vi "IV analysis.vi"() -> ()   [LabVIEW 2020]
uses:
  <userlib>/Levylab/LV to ITX/Data/Typedefs/File Type--enum.ctl
  <userlib>/Levylab/XY Utilities/subVIs/Savitsky Golay Filter (single).vi
  <userlib>/Levylab/XY Utilities/subVIs/Difference Quotient (single).vi
  <userlib>/Levylab/XY Utilities/xy_utilities.lvlib
  data-analysis-megan/Retrieve and Visualize/Retrieve and Visualize.lvclass
  <userlib>/Levylab/LV to ITX/Data/Data.lvclass
panel:
  in  "start (length of curve)":i32
  in  "length of curve":i32
  in  "side points 2T":i32
  in  "side points 4T":i32
  in  "Interval Units":enum16{"Points", "Data"}(ring)
  in  "Window [h]":dbl=250.0 min=2.0
  in  "Tab Control":T1(tab)
  in  "index":T2
  in  "File or Folder Path":path=path "C:/Users/voodoo/Desktop/IV_separat_Vsgsweep_2fields_Vbg-2.8V"
  in  "decimate files":i32=1
  in  "offset":i32
  in  "length":i32=1
  in  "File Type":T3
  out "Comments":string="Device: \r  Device Name: SA40178.20210125\r  Computer: KHOLEK\r  User: Aditi\r  Instrument: MNK\r  Description: |\r        devices:\r        \r        1. 80x80um rectangle\r        2. hash: 200 horizontal and vertical lines 400nm apart\r        3. hash structures: 400, 200nm apart horizontal and vertical lines\r\rExperiment: \r  Time: 2021-02-01T16:02:55\r  Description: |\r     IV measurements at 0T\r     - Sweep priority 0: +x gate from -10V to 10V in steps of 1V (-x 10 to -10)\r     - priority 1:+y gate from -10V to 10V in steps of 1V (-y 10 to -10)\r    - 5s wait\r     - 1 IV curves at each Vsg\r     - KH channel 17,18,19,20: leads 3,8,15,27\r    Vbg = lead 26: 0V\r    T: 20mK\r    \r    \r    400nm periodicity mesh\r    \r    KH channel 2,1: leads 5,4 , current mode, 5k resistor, 1000x gain\r    lead 5: 10mV ac+ 0uV dc bias, 0.02 Hz\r    KH channel 3,4: V1+/-: 6,7 1000x gain\r    \r    rectangle\r    \r    KH channel 5,8: leads 9,13 , current mode, 5k resistor, 1000x gain\r     lead 9: 10mV ac+ 0uV dc bias, 0.02 Hz\r     KH channel 6,7: V1+/-: 11,12 1000x gain\r    \r    \r    200nm periodicity mesh\r    \r    KH channel 12,11: leads 21,20 , current mode, 5k resistor, 1000x gain\r    lead 21: 10mV ac+ 180uV dc bias, 0.02 Hz\r    KH channel 9,10: V1+/-: 16,17 1000x gain\r    \r    line filter on in lockin\r    decimating factor: 5\r\rSweep: \r- Loop1: [Lockin Bias, 10.000000]\r- Loop2: [Lockin Bias, 10.000000]\r- Loop3: [OFF, 0.000000]\r- Loop4: [OFF, 0.000000]\r\rWiring: \r- Electrode 4: Lockin 1, I2, KH1 Channel 1, Differential, 1000x, 5k Ohms\r- Electrode 5: Lockin 2, I2, KH1 Channel 2, Differential, 1000x, 5k Ohms\r- Electrode 6: Lockin 3, V2, KH1 Channel 3, SE+ (-gnd), 1000x, Open\r- Electrode 7: Lockin 4, V2, KH1 Channel 4, SE+ (-gnd), 1000x, Open\r- Electrode 9: Lockin 5, I2, KH1 Channel 5, Differential, 1000x, 5k Ohms\r- Electrode 11: Lockin 6, V2, KH1 Channel 6, SE+ (-gnd), 1000x, Open\r- Electrode 12: Lockin 7, V2, KH1 Channel 7, SE+ (-gnd), 1000x, Open\r- Electrode 13: Lockin 8, I2, KH1 Channel 8, Differential, 1000x, 5k Ohms\r- Electrode 16: Lockin 9, V1+, KH2 Channel 1, SE+ (-gnd), 1000x, Open\r- Electrode 17: Lockin 10, V1-, KH2 Channel 2, SE+ (-gnd), 1000x, Open\r- Electrode 20: Lockin 11, I-, KH2 Channel 3, Differential, 1000x, 5k Ohms\r- Electrode 21: Lockin 12, I+, KH2 Channel 4, Differential, 1000x, 5k Ohms\r- Electrode 1: Lockin 13, Vsg, KH2 Channel 5, Differential, 1000x, 50k Ohms\r\rLockin: \r  AO: \r  - AO 1: amp = 0.000 mV, DC = 0.000 mV, f = 0.02 Hz, phi = 0.00°, Triangle\r  - AO 2: amp = 10.000 mV, DC = 0.000 mV, f = 0.02 Hz, phi = 0.00°, Triangle\r  - AO 3: amp = 0.000 mV, DC = 0.000 mV, f = 0.02 Hz, phi = 0.00°, Triangle\r  - AO 4: amp = 0.000 mV, DC = 0.000 mV, f = 0.02 Hz, phi = 0.00°, Triangle\r  - AO 5: amp = 10.000 mV, DC = 0.000 mV, f = 0.02 Hz, phi = 0.00°, Triangle\r  - AO 6: amp = 0.000 mV, DC = 0.000 mV, f = 0.02 Hz, phi = 0.00°, Triangle\r  - AO 7: amp = 0.000 mV, DC = 0.000 mV, f = 0.02 Hz, phi = 0.00°, Triangle\r  - AO 8: amp = 0.000 mV, DC = 0.000 mV, f = 0.02 Hz, phi = 0.00°, Triangle\r  - AO 9: amp = 0.000 mV, DC = 0.000 mV, f = 0.02 Hz, phi = 0.00°, Triangle\r  - AO 10: amp = 0.000 mV, DC = 0.000 mV, f = 0.02 Hz, phi = 0.00°, Triangle\r  - AO 11: amp = 0.000 mV, DC = 0.000 mV, f = 0.02 Hz, phi = 0.00°, Triangle\r  - AO 12: amp = 10.000 mV, DC = 0.180 mV, f = 0.02 Hz, phi = 0.00°, Triangle\r  - AO 13: amp = 0.000 mV, DC = 0.000 mV, f = 0.02 Hz, phi = 0.00°, Sine\r  - AO 14: amp = 0.000 mV, DC = 0.000 mV, f = 0.02 Hz, phi = 0.00°, Sine\r  - AO 15: amp = 0.000 mV, DC = 0.000 mV, f = 0.02 Hz, phi = 0.00°, Sine\r  - AO 16: amp = 0.000 mV, DC = 0.000 mV, f = 0.02 Hz, phi = 0.00°, Sine\r  - AO 17: amp = 0.000 mV, DC = -10000.000 mV, f = 0.02 Hz, phi = 0.00°, Sine\r  - AO 18: amp = 0.000 mV, DC = -10000.000 mV, f = 0.02 Hz, phi = 0.00°, Sine\r  - AO 19: amp = 0.000 mV, DC = 10000.000 mV, f = 0.02 Hz, phi = 0.00°, Sine\r  - AO 20: amp = 0.000 mV, DC = 10000.000 mV, f = 0.02 Hz, phi = 0.00°, Sine\r  - AO 21: amp = 0.000 mV, DC = 0.000 mV, f = 0.02 Hz, phi = 0.00°, Sine\r  - AO 22: amp = 0.000 mV, DC = 0.000 mV, f = 0.02 Hz, phi = 0.00°, Sine\r  - AO 23: amp = 0.000 mV, DC = 0.000 mV, f = 0.02 Hz, phi = 0.00°, Sine\r  - AO 24: amp = 0.000 mV, DC = 0.000 mV, f = 0.02 Hz, phi = 0.00°, Sine\r  REF: \r  - Lockin 1: f = 0.02 Hz, phi = 0.00°, TC = 0.10 s, order = 2 \r  Sampling: \r  - Fs: 1000.000000\r  - N: 50000\r"
  out "Gates and B":T4
  out "Common Mode":cluster{dbl[], dbl[]}(graph)
  out "Differential mode":cluster{dbl[], dbl[]}(graph)
  out "V2T vs I":cluster{dbl[], dbl[]}[](graph)
  out "V4T vs I":cluster{dbl[], dbl[]}[](graph)
  out "G2T vs V2T":cluster{"Array out":dbl[], "Array out":dbl[]}[](graph)
  out "R2T vs I":cluster{"Array out":dbl[], "Array out":dbl[]}[](graph)
  out "R4T vs I":cluster{"Array out":dbl[], "Array out":dbl[]}[](graph)
  out "G4T vs V4T":cluster{"Array out":dbl[], "Array out":dbl[]}[](graph)
  out "R2T":dbl[][](graph)
  out "R4T":dbl[][](graph)
  # "Analysis controls"
  # "S-G filter"
  # "Derivative parameters"
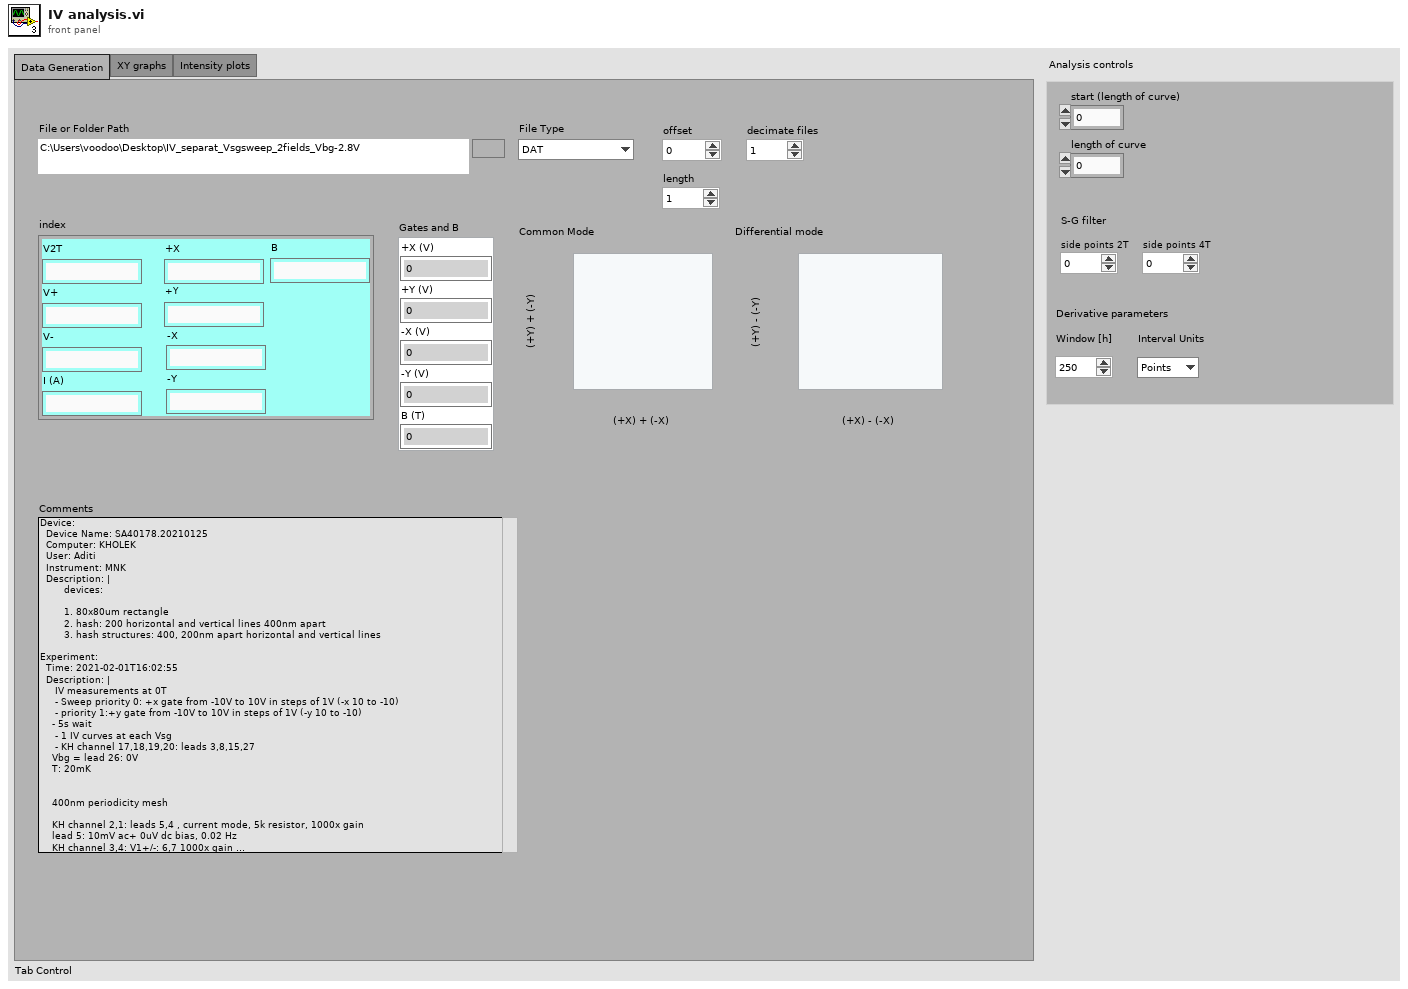
[diagram p1: front panel]
types:
  T1 = enum32{"Data Generation", "XY graphs", "Intensity plots"}
  T2 = cluster{"V2T":string, "V+":string, "V-":string, "I (A)":string, "+X":string, "+Y":string, "-X":string, "-Y":string, "B":string}
  T3 = typedef "Data.lvclass/File Type--enum.ctl" = enum16{"DAT", "ITX", "TDMS", "VI"}
  T4 = cluster{"+X (V)":dbl, "+Y (V)":dbl, "-X (V)":dbl, "-Y (V)":dbl, "B (T)":dbl}
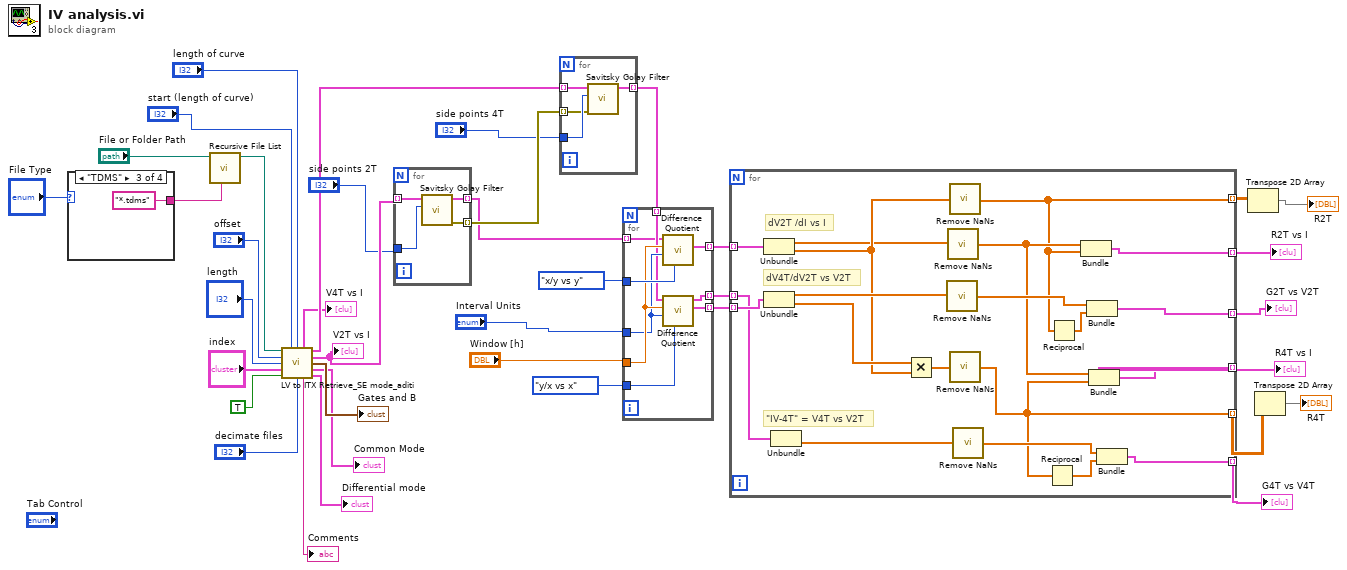
[diagram p0: block diagram]
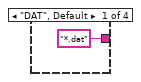
[diagram p2: hidden frame]
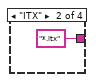
[diagram p3: hidden frame]
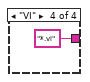
[diagram p4: hidden frame]
diagram:
  n1 = case shown="\"TDMS\"" "File Type" {
    tunnel: ["*.dat" ("pattern") "*.itx" ("pattern") "*.tdms" ("pattern") "*.vi" ("pattern")] -> w22
    frame "DAT", Default {
    }
    frame "ITX" {
    }
    frame "TDMS" {
    }
    frame "VI" {
    }
  }
  n2 = call <vilib>:"Recursive File List.vi"("pattern"=w22, "Folder Path"="File or Folder Path") -> ("dup Folder Path"=w24:path)  [unwired: 5 in, 4 out]
  n3 = call "LV to ITX Retrieve_SE mode_aditi.vi"("File or Folder Path"=w24, "start"="start (length of curve)", 2:"length"="length of curve", "offset"="offset", 7:"length"="length", "index"="index", "stop"=TRUE, "decimate files"="decimate files") -> ("I-V4T"=→"V4T vs I":cluster{dbl[], dbl[]}[], "V2T-V4T"=w14:cluster{dbl[], dbl[]}[], "V2T-I"=w15:cluster{dbl[], dbl[]}[], "Gates and B"=→"Gates and B":T4, "Common Mode"=→"Common Mode":cluster{dbl[], dbl[]}, "Comments"=→"Comments":string, "Differential mode"=→"Differential mode":cluster{dbl[], dbl[]})  [unwired: 1 in]
  "V2T vs I" <- w15
  n4 = for {
    tunnel: "side points 2T" -> [w45]
    tunnel: [w46] -> w16 mode=indexing
    tunnel: w15 -> [w44] mode=indexing
    tunnel: [w43] -> w18 mode=indexing
    n5 = call-poly <userlib>:"Savitsky Golay Filter.vi"("side points"=w45, "XY-data"=w44) -> ("error out"=w43:errorcluster, "XY-data out"=w46:cluster{"X-array":dbl[], "Y-array":dbl[]})  [unwired: 8 in]
  }
  n6 = for {
    tunnel: "side points 4T" -> [w50]
    tunnel: w14 -> [w49] mode=indexing
    tunnel: w18 -> [w48] mode=indexing
    tunnel: [w47] -> w17 mode=indexing
    n7 = call-poly <userlib>:"Savitsky Golay Filter.vi"("error in (no error)"=w48, "side points"=w50, "XY-data"=w49) -> ("XY-data out"=w47:cluster{"X-array":dbl[], "Y-array":dbl[]})  [unwired: 7 in, 1 out]
  }
  n8 = for {
    tunnel: enum16{"y/x vs x", "x/y vs y"}."x/y vs y" ("Type 2") -> [w59]
    tunnel: [w57] -> w34 mode=indexing
    tunnel: "Window [h]" -> [w56]
    tunnel: "Interval Units" -> [w55]
    tunnel: enum16{"y/x vs x", "x/y vs y"}."y/x vs x" ("Type 2") -> [w54]
    tunnel: [w53] -> w32 mode=indexing
    tunnel: [w58] -> w35 mode=indexing
    tunnel: w17 -> [w52] mode=indexing
    tunnel: w16 -> [w51] mode=indexing
    n9 = call-poly <userlib>:"Difference Quotient.vi"("Type"=w59, "Interval Units (points)"=w55, "Window [h] (2)"=w56, "XY-data"=w51) -> ("Difference Quotient"=w58:cluster{"X-array":dbl[], "Y-array":dbl[]})  [unwired: 5 in, 2 out]
    n10 = call-poly <userlib>:"Difference Quotient.vi"("Type"=w54, "Interval Units (points)"=w55, "Window [h] (2)"=w56, "XY-data"=w52) -> ("Difference Quotient"=w57:cluster{"X-array":dbl[], "Y-array":dbl[]}, "XY-data out"=w53:cluster{"X-array":dbl[], "Y-array":dbl[]})  [unwired: 5 in, 1 out]
  }
  n11 = for {
    tunnel: [w79] -> w27 mode=indexing
    tunnel: [w78] -> w38 mode=indexing
    tunnel: [w77] -> w26 mode=indexing
    tunnel: [w76] -> w37 mode=indexing
    tunnel: w35 -> [w75] mode=indexing
    tunnel: w34 -> [w74] mode=indexing
    tunnel: w32 -> [w73] mode=indexing
    tunnel: [w61] -> w31 mode=indexing
    tunnel: [w62] -> w30 mode=indexing
    # "dV2T /dI vs I"
    # "dV4T/dV2T vs V2T"
    # "\"IV-4T\" = V4T vs V2T"
    n12 = Unbundle(w75) -> ("X-array"=w67:dbl[], "Y-array"=w69:dbl[])
    n13 = Unbundle(w74) -> ("X-array"=w70:dbl[], "Y-array"=w71:dbl[])
    n14 = Unbundle(w73) -> ("Y-array"=w72:dbl[])  [unwired: 1 out]
    n15 = Multiply(x=w71, y=w69) -> (x*y=w64:dbl[])
    n16 = call "Remove NaNs.vi"("Array in"=w70) -> ("Array out"=w68:dbl[])
    n17 = call "Remove NaNs.vi"("Array in"=w67) -> ("Array out"=w65:dbl[])
    n18 = call "Remove NaNs.vi"("Array in"=w69) -> ("Array out"=w62:dbl[])
    n19 = call "Remove NaNs.vi"("Array in"=w64) -> ("Array out"=w61:dbl[])
    n20 = call "Remove NaNs.vi"("Array in"=w72) -> ("Array out"=w66:dbl[])
    n21 = Reciprocal(x=w61) -> (1/x=w60:dbl[])
    n22 = Reciprocal(x=w62) -> (1/x=w63:dbl[])
    n23 = Bundle("Array out"=w65, "Array out"=w62) -> (w78:cluster{"Array out":dbl[], "Array out":dbl[]})  [unwired: 1 in]
    n24 = Bundle("Array out"=w68, w63) -> (w79:cluster{"Array out":dbl[], dbl[]})  [unwired: 1 in]
    n25 = Bundle("Array out"=w65, "Array out"=w61) -> (w76:cluster{"Array out":dbl[], "Array out":dbl[]})  [unwired: 1 in]
    n26 = Bundle("Array out"=w66, w60) -> (w77:cluster{"Array out":dbl[], dbl[]})  [unwired: 1 in]
  }
  "R4T vs I" <- w37
  "G4T vs V4T" <- w26
  "R2T vs I" <- w38
  "G2T vs V2T" <- w27
  n27 = Transpose 2D Array(2D array=w30) -> (transposed array=→"R2T":dbl[][])
  n28 = Transpose 2D Array(2D array=w31) -> (transposed array=→"R4T":dbl[][])
